vi "IPVoice.FRAME_RD.vi"(0 "VISA resource name":refnum<visa-resource-name> caption="Serial Port", 1 "timeout(ms)":u32=5000 caption="超时（ms）", 11 "error in (no error)":errorcluster caption="错误输入（无错误）", 12 "字节总数":u32) -> (4 "OK?":bool, 10 "返回数组":i32[][](array[numeric]) format="%02x", 14 "返回数":u32, 15 "error out":errorcluster caption="错误输出")   [LabVIEW 2012, in "Lib_UEL.ATE.lvlib" / "Lib_IPVoice.lvlib"]
uses:
  Lib_IPVoice.lvlib
  <vilib>/Instr/_visa.llb/VISA Configure Serial Port (Instr).vi
panel:
  in  "baud rate (9600)":u32=9600 caption="波特率(9600)"
  # "V001 - Inital Version. ~Nick 2015-01-08"
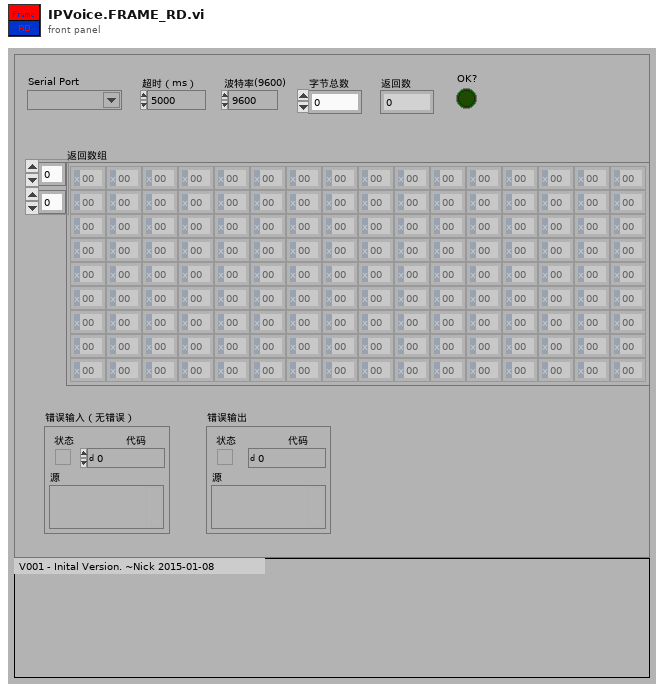
[diagram p1: front panel]
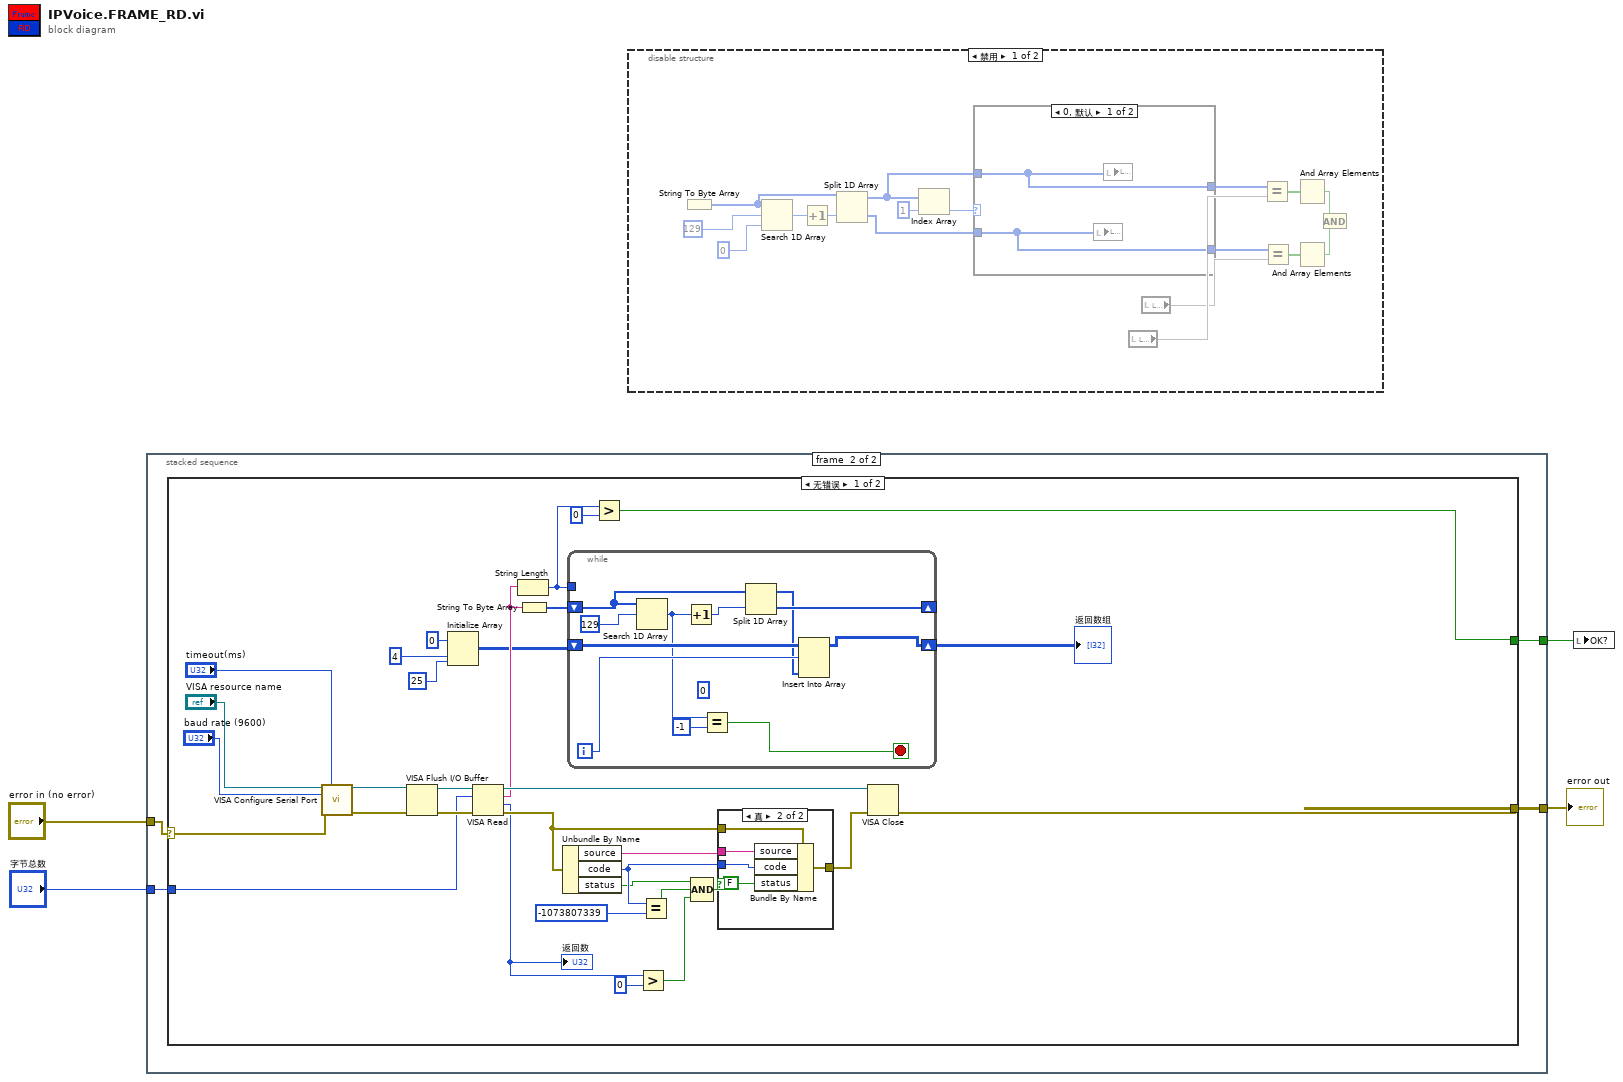
[diagram p0: block diagram]
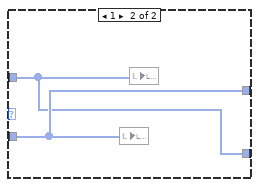
[diagram p2: hidden frame]
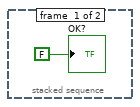
[diagram p4: hidden frame]
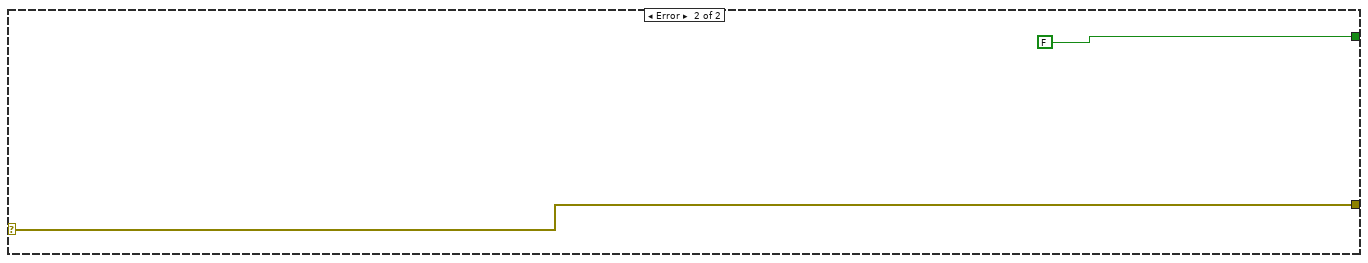
[diagram p6: hidden frame]
diagram:
  n1 = stacked-sequence {
    tunnel: "error in (no error)" -> [_ w9]
    tunnel: [_ w8] -> w3
    tunnel: "字节总数" -> [_ w7]
    tunnel: [_ w6] -> w1
    frame #0 {
      "OK?" <- FALSE ("OK?")
    }
    frame #1 {
      n2 = case shown="无错误" w9 {
        selector: w9 -> [w38 w60]
        tunnel: [w36 w60] -> w8
        tunnel: w7 -> [w14 _]
        tunnel: [w17 FALSE] -> w6
        frame No Error {
          n3 = call-poly "VISA Configure Serial Port"("VISA resource name"="VISA resource name", "timeout (10sec)"="timeout(ms)", "baud rate (9600)"="baud rate (9600)", "error in (no error)"=w38) -> ("VISA resource name out"=w35:refnum<visa-resource-name>, "error out"=w34:errorcluster)  [unwired: 10 in]
          n4 = VISA Flush I/O Buffer(VISA resource name=w35, error in (no error)=w34) -> (VISA resource name out=w33:refnum<visa-resource-name>, error out=w32:errorcluster)  [unwired: 1 in]
          n5 = Initialize Array(u8 0 ("元素"), 4 ("维数大小"), 25 ("维数大小")) -> (w13:u8[][])
          n6 = VISA Read(VISA resource name=w33, byte count=w14, error in (no error)=w32) -> (VISA resource name out=w37:refnum<visa-resource-name>, read buffer=w19:string, return count=w23:u32, error out=w30:errorcluster)
          "返回数" <- w23
          n7 = String Length(string=w19) -> (length=w16:i32)
          n8 = String To Byte Array(string=w19) -> (unsigned byte array=w18:u8[])
          n9 = Unbundle By Name(w30) -> ("source"=w29:string, "code"=w28:i32, "status"=w25:bool)
          n10 = while {
            shift-right: [w50] -> _
            shift-left: w18 -> [w51]
            shift-right: [w46] -> w15
            shift-left: w13 -> [w47]
            tunnel: w16 -> [_]
            i -> [w48]
            stop <- w42 stop-if-true
            (unwired) 0 ("禁用的索引 (列)")
            n11 = Search 1D Array(1D array=w51, element=u8 129 ("元素")) -> (index of element=w44:i32)  [unwired: 1 in]
            n12 = Increment(x=w44) -> (x+1=w49:i32)
            n13 = Equal?(x=w44, y=-1) -> (x = y?=w42:bool)
            n14 = Split 1D Array(array=w51, index=w49) -> (first subarray=w45:u8[], second subarray=w50:u8[])
            n15 = Insert Into Array(array=w47, index (row)=w48, new element=w45) -> (w46:u8[][])  [unwired: 1 in]
          }
          "返回数组" <- w15
          n16 = Greater?(x=w16, y=0) -> (0:w17:bool)
          n17 = Greater?(x=w23, y=u32 0) -> (0:w21:bool)
          n18 = Equal?(x=w28, y=-1073807339) -> (x = y?=w26:bool)
          n19 = Compound Arithmetic op=AND(w25, w26, w21) -> (w24:bool)
          n20 = case shown="真" w24 {
            tunnel: w30 -> [w53 w58]
            tunnel: w29 -> [_ w57]
            tunnel: w28 -> [_ w56]
            tunnel: [w53 w54] -> w27
            frame False {
            }
            frame True {
              n21 = Bundle By Name(cluster=w58, "source"=w57, "code"=w56, "status"=FALSE) -> (w54:errorcluster)
            }
          }
          n22 = VISA Close(VISA resource name=w37, error in (no error)=w27) -> (error out=w36:errorcluster)
        }
        frame Error {
        }
      }
    }
  }
  "error out" <- w3
  n23 = disable-structure shown="禁用" {
    frame Disabled {
      n24 = String To Byte Array() -> (unsigned byte array=w63:u8[])  [unwired: 1 in]
      n25 = Search 1D Array(1D array=w63, element=u8 129 ("元素"), start index (0)=0 ("开始索引(0)")) -> (index of element=w77:i32)
      n26 = Increment(x=w77) -> (x+1=w76:i32)
      n27 = Split 1D Array(array=w63, index=w76) -> (first subarray=w66:u8[], second subarray=w67:u8[])
      n28 = Index Array(array=w66, index=1 ("索引")) -> (element=w65:u8)
      n29 = case shown="0, 默认" w65 {
        tunnel: w66 -> [w79 w80]
        tunnel: w67 -> [w78 w81]
        tunnel: [w79 w81] -> w70
        tunnel: [w78 w80] -> w68
        frame 0, Default {
          n30 = local write item#-1(w78) -> ()
          n31 = local write item#-1(w79) -> ()
        }
        frame 1 {
          n32 = local write item#-1(w81) -> ()
          n33 = local write item#-1(w80) -> ()
        }
      }
      n34 = local read item#-1() -> (w71)
      n35 = local read item#-1() -> (w69)
      n36 = Equal?(x=w70, y=w71) -> (x = y?=w72:bool[])
      n37 = Equal?(x=w68, y=w69) -> (x = y?=w73:bool[])
      n38 = And Array Elements(Boolean array=w72) -> (logical AND=w74:bool)
      n39 = And Array Elements(Boolean array=w73) -> (logical AND=w75:bool)
      n40 = And(x=w74, y=w75) -> ()  [unwired: 1 out]
    }
    frame Enabled {
    }
  }
  n41 = local write "OK?"(w1) -> ()
